vi "Encoder_Sentido.vi"() -> ()   [LabVIEW 2025]
panel:
  in  "Restablecer conteo":bool
  out "Conteo":dbl
  in  "stop":bool
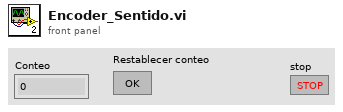
[diagram p1: front panel]
types:
  T1 = enum16{"Inicio", "L1", "L2", "L3", "Restar", "R1", "R2", "R3", "Sumar", ""}
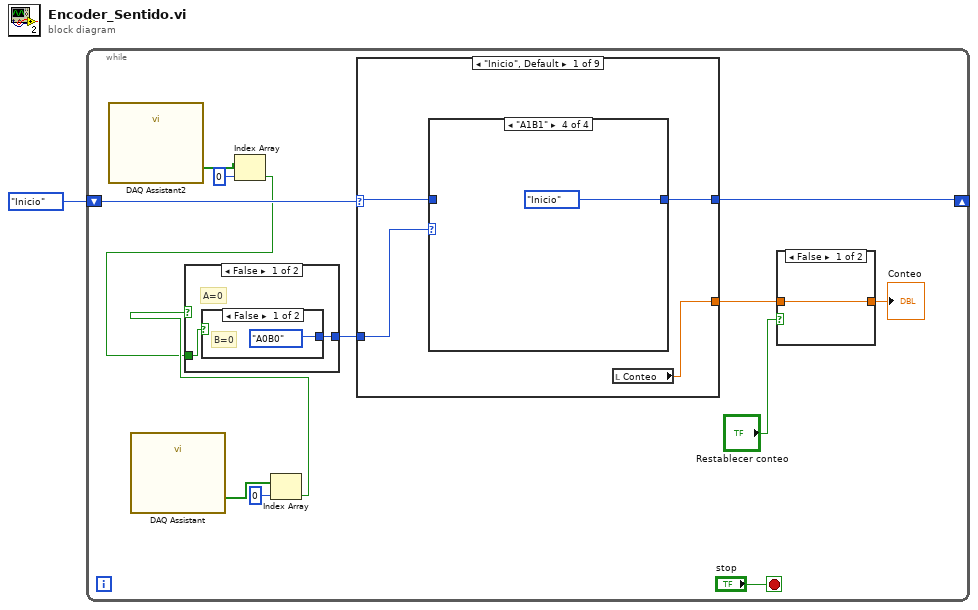
[diagram p0: block diagram]
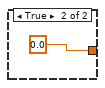
[diagram p2: hidden frame]
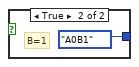
[diagram p3: hidden frame]
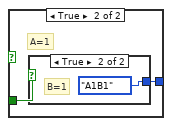
[diagram p4: hidden frame]
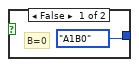
[diagram p5: hidden frame]
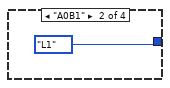
[diagram p7: hidden frame]
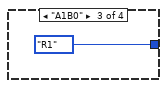
[diagram p8: hidden frame]
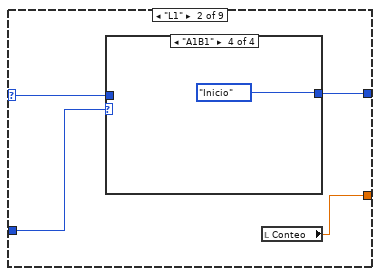
[diagram p9: hidden frame]
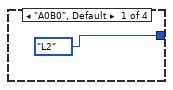
[diagram p10: hidden frame]
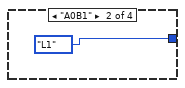
[diagram p11: hidden frame]
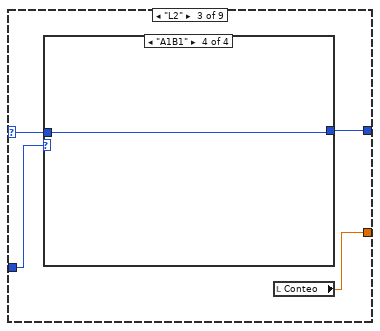
[diagram p13: hidden frame]
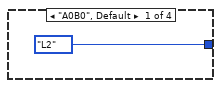
[diagram p14: hidden frame]
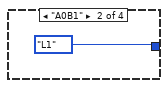
[diagram p15: hidden frame]
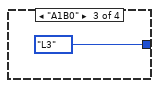
[diagram p16: hidden frame]
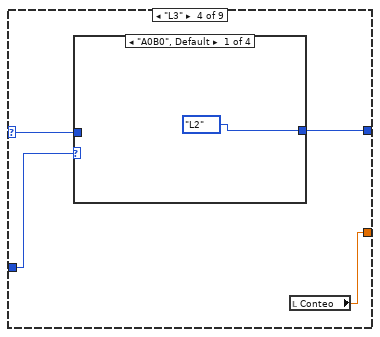
[diagram p17: hidden frame]
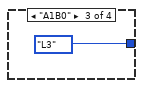
[diagram p19: hidden frame]
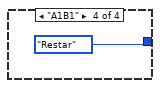
[diagram p20: hidden frame]
diagram:
  n1 = while {
    shift-right: [w11] -> _
    shift-left: T1."Inicio" -> [w14]
    stop <- "stop" stop-if-true
    n2 = call "DAQ Assistant2"() -> ("data"=w4:bool[])  [unwired: 17 in, 2 out]
    n3 = call "DAQ Assistant"() -> ("data"=w7:bool[])  [unwired: 17 in, 2 out]
    n4 = Index Array(array=w4, index=0) -> (element=w2:bool)
    n5 = Index Array(array=w7, index=0) -> (element=w5:bool)
    n6 = case shown="False" w5 {
      tunnel: [w18 w22] -> w13
      tunnel: w2 -> [w17 w21]
      frame False {
        # "A=0"
        n7 = case shown="False" w17 {
          tunnel: [enum16{"A0B0", "A0B1", "A1B0", "A1B1"}."A0B0" enum16{"A0B0", "A0B1", "A1B0", "A1B1"}."A0B1"] -> w18
          frame False {
            # "B=0"
          }
          frame True {
            # "B=1"
          }
        }
      }
      frame True {
        # "A=1"
        n8 = case shown="True" w21 {
          tunnel: [enum16{"A0B0", "A0B1", "A1B0", "A1B1"}."A1B0" enum16{"A0B0", "A0B1", "A1B0", "A1B1"}."A1B1"] -> w22
          frame False {
            # "B=0"
          }
          frame True {
            # "B=1"
          }
        }
      }
    }
    n9 = case shown="\"Inicio\", Default" w14 {
      selector: w14 -> [w26 w34 w42 w50 _ w60 w68 w76 _]
      tunnel: w13 -> [w28 w36 w44 w52 _ w62 w70 w78 _]
      tunnel: [w27 w35 w43 w51 T1."Inicio" w61 w69 w77 T1."Inicio"] -> w11
      tunnel: [w25 w33 w41 w49 w57 w63 w71 w79 w85] -> w8
      frame "Inicio", Default {
        n10 = case shown="\"A1B1\"" w28 {
          tunnel: [w29 T1."L1" T1."R1" T1."Inicio"] -> w27
          tunnel: w26 -> [w29 _ _ _]
          frame "A0B0", Default {
          }
          frame "A0B1" {
          }
          frame "A1B0" {
          }
          frame "A1B1" {
          }
        }
        n11 = local read "Conteo"() -> (w25:dbl)
      }
      frame "L1" {
        n12 = case shown="\"A1B1\"" w36 {
          tunnel: [T1."L2" T1."L1" w39 T1."Inicio"] -> w35
          tunnel: w34 -> [_ _ w39 _]
          frame "A0B0", Default {
          }
          frame "A0B1" {
          }
          frame "A1B0" {
          }
          frame "A1B1" {
          }
        }
        n13 = local read "Conteo"() -> (w33:dbl)
      }
      frame "L2" {
        n14 = case shown="\"A1B1\"" w44 {
          tunnel: [T1."L2" T1."L1" T1."L3" w48] -> w43
          tunnel: w42 -> [_ _ _ w48]
          frame "A0B0", Default {
          }
          frame "A0B1" {
          }
          frame "A1B0" {
          }
          frame "A1B1" {
          }
        }
        n15 = local read "Conteo"() -> (w41:dbl)
      }
      frame "L3" {
        n16 = case shown="\"A0B0\", Default" w52 {
          tunnel: [T1."L2" w54 T1."L3" T1."Restar"] -> w51
          tunnel: w50 -> [_ w54 _ _]
          frame "A0B0", Default {
          }
          frame "A0B1" {
          }
          frame "A1B0" {
          }
          frame "A1B1" {
          }
        }
        n17 = local read "Conteo"() -> (w49:dbl)
      }
      frame "Restar" {
        n18 = local read "Conteo"() -> (w58:dbl)
        n19 = Decrement(x=w58) -> (x-1=w57:dbl)
      }
      frame "R1" {
        n20 = case shown="\"A1B1\"" w62 {
          tunnel: [T1."R2" w65 T1."R1" T1."Inicio"] -> w61
          tunnel: w60 -> [_ w65 _ _]
          frame "A0B0", Default {
          }
          frame "A0B1" {
          }
          frame "A1B0" {
          }
          frame "A1B1" {
          }
        }
        n21 = local read "Conteo"() -> (w63:dbl)
      }
      frame "R2" {
        n22 = case shown="\"A0B0\", Default" w70 {
          tunnel: [T1."R2" T1."R3" T1."R1" w75] -> w69
          tunnel: w68 -> [_ _ _ w75]
          frame "A0B0", Default {
          }
          frame "A0B1" {
          }
          frame "A1B0" {
          }
          frame "A1B1" {
          }
        }
        n23 = local read "Conteo"() -> (w71:dbl)
      }
      frame "R3" {
        n24 = case shown="\"A1B0\"" w78 {
          tunnel: [T1."R2" T1."R3" w82 T1."Sumar"] -> w77
          tunnel: w76 -> [_ _ w82 _]
          frame "A0B0", Default {
          }
          frame "A0B1" {
          }
          frame "A1B0" {
          }
          frame "A1B1" {
          }
        }
        n25 = local read "Conteo"() -> (w79:dbl)
      }
      frame "Sumar" {
        n26 = local read "Conteo"() -> (w86:dbl)
        n27 = Increment(x=w86) -> (x+1=w85:dbl)
      }
    }
    n28 = case shown="False" "Restablecer conteo" {
      tunnel: [w15 0.0 ("Conteo")] -> w9
      tunnel: w8 -> [w15 _]
      frame False {
      }
      frame True {
      }
    }
    "Conteo" <- w9
  }
